vi "FestoCPX.Station.Prod.DropNOK.vi"(7 "prev status":T1=enum."Error", 8 "error in":errorcluster, 10 "Serial":i32, 11 "Slot":T3) -> (0 "error out":errorcluster, 1 "Pause status":T2, 2 "Final status":T1)   [LabVIEW 2016]
uses:
  Station/Station.ProductSlot.ctl
  Sequence/Sequence.Step.Status.ctl
  Sequence/Sequence.Test.BreakReason.ctl
  tools/Translator/Translator.Message.ctl
  tools/EventLog/EventLog.EventSource.ctl
  Station/Station.ValvePosition.ctl
  tools/EventLog/EventLog.CreateError(single).vi
  tools/EventLog/EventLog.New(array).vi
  Sequence/Sequence.SerialsFglb.Action.ctl
  Sequence/Sequence.SerialsFglb.SerialData.ctl
  Global/ApplicationGlobal.vi
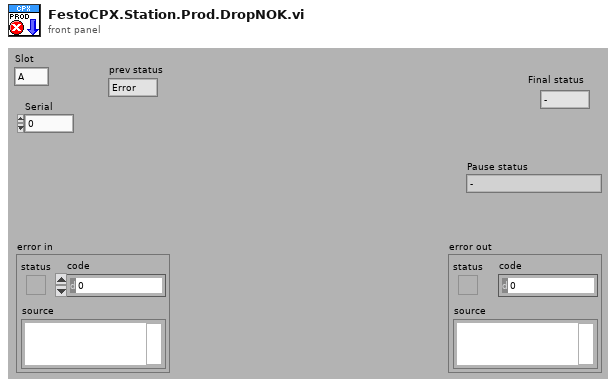
[diagram p1: front panel]
types:
  T1 = typedef "Sequence.Step.Status.ctl" = enum16{"-", "Pending", "Running", "Skipped", "Passed", "Failed", "Done", "Error", "Aborted", "Stopped"}
  T2 = typedef "Sequence.Test.BreakReason.ctl" = enum16{"-", "NOK container", "OK container", "Rev empty", "Rev missing", "Rev wrong", "Fork missing", "Fork wrong", "NOK limit", "Unload failure", "Single slot", "Part done", "Err: Prod move work", "Err: Prod move home", "Err: Prod lift work", "Err: Prod lift home", "Err: Prod Arm Work", "Err: Prod Arm NOK", "Err: Prod Arm OK", "Err: Prod NOK suck", "Err: Prod NOK drop", "Err: Prod OK missing", "Err: Prod OK suck", "Err: Prod OK drop"}
  T3 = typedef "Station.ProductSlot.ctl" = enum8{"A", "B"}
  T4 = typedef "Translator.Message.ctl" = enum16{"-", "Event confirmed", "Log out", "Log in", "Shutdown", "Cancel", "Start", "Begin time", "End time", "Duration", "Service Mode", "Ignore Results", "Serial Format", "On", "Off", "OK", "NOK", "NOK %s", "Home", "Work", "Close", "Open", "In progress...", "Missing", "Empty", "Hardware failure", "Initial", "Default", "Total", "Out of range", "Free disk space is below 1GB - contact technician", "Error %d >> %s", "Error %d >> %s >> %s", "Msg %d >> %s", "Laser msg %d %s", "Laser cmd error %s %d", "Laser cmd failed %s", "Laser cmd warning %s", "Laser disconnected", "Laser status %s", "Laser already started", "Laser job unkonwn %s", "Laser job missing %s", "Laser job select failure %s", "Unable to start laser printing (%s)", "Unable to stop laser printing (%s)", "Laser marking aborted", "Laser marking timeout", "Unable to reset Laser Interlock (%s)", "Unable to trigger Laser. Laser not ready (%s)", "Laser job '%s' coordinates not configured", "Starting %s", "Quitting %s", "Configured", "Initializing", "Quitting", "Loading", "Loaded %d results", "Loaded %d events", "Running", "Stopped", "Summary", "Laser", "Do you want to continue?", "Do you want to delete the configuration?", "The configuration is being used by an order. Unable to delete!", "Press confirm button", "Station is not based. Do you want to exit?", "Station requires changeover. Do you want to run the test?", "Test options are not set as default. Do you want to continue?", "Formatting of WabcoNo is disabled. Do you want to continue?", "Product not detected. Do you want to continue?", "Product scan failed. Do you want to continue?", "Calibration", "Log out?", "System", "All", "IDLE", "Translating...%s", "Not found", "Alarm %s", "Run", "Skip", "Abort", "Repeat", "Please wait...", "Database disconnected", "Database disconnected - changeover disabled!", "Login to database successful", "Login to database failed: %d; %s", "Unable to check the product status of reference %d - database disconnected", "Unable to set the product status of reference %d - database disconnected", "Variant file backup %s", "Read variant (%s)", "Result", "Station armed!", "Station requires changeover!", "Select reference number...", "EMERGENCY BUTTON - press Control button", "EMERGENCY DOOR - press Control button", "Resetting Emergency...", "Unable to reset safety circuit - Emergency Button pressed", "Unable to reset safety circuit - Emergency Side Door open", "Station not based", "Station based", "Station not empty", "Station basing...", "No order", "Press Start to begin new order", "Scanning new order", "Order NOK. Correct or scan again", "Order OK. Press Accept", "Order ready", "Revolver incorrect", "Fork incorrect", "Revolver missing", "Revolver empty", "Container missing", "Offline results", "Offline statistics", "Updating statistics %.1f %%", "DMC Configurator", "Door open", "Close the front door", "Press start button", "Done. Open the front door", "Running...", "Running...%.1f %%", "Pause %s", "Pause %s. NOK container missing", "Pause %s. OK container missing", "Pause %s. Revolver empty", "Pause %s. Revolver missing", "Pause %s. Revolver incorrect", "Pause %s. Fork missing", "Pause %s. Fork incorrect", "Pause %s. Too many failures", "Pause %s. Unloading failure", "Pause %s. One slot is not working", "Pause %s. Part order is done. Empty OK container", "Pause %s. Unable to move product to slot", "Pause %s. Unable to move back product pusher", "Pause %s. Unable to lift product", "Pause %s. Unable to move back product lifter", "Pause %s. Unable to move product arm to Work", "Pause %s. Unable to move product arm to NOK", "Pause %s. Unable to move product arm to OK", "Pause %s. Unable to unsuck the NOK product", "Pause %s. Unable to drop the NOK product", "Pause %s. Product OK missing", "Pause %s. Unable to unsuck the OK product", "Pause %s. Unable to drop the OK product", "Stopping...", "File '%s' is missing", "File '%s' is broken", "File '%s' is running", "Log file started (%s)", "Log file ended (%s)", "Log file stopped (%s)", "Log file ignored (%s)", "Log file exported (%s)", "Log file export failed (%s)", "Wrong serial number in log file", "Wrong reference number in log file", "Test steps are missing", "%s = %.3f", "Process param '%s' not found in DB", "Process param '%s' wrong order", "Process param '%s' value %.3f out of limits (%.3f; %.3f)", "Step%d param '%s' not found in DB", "Step%d param '%s' wrong order", "Step%d param '%s' value %.3f out of limits (%.3f; %.3f)", "Step%d EV '%s' not found in DB", "Step%d EV '%s' wrong order", "\"%s\" not found in DB", "\"%s\" wrong order", "\"%s\" value %.3f out of limits (%.3f; %.3f)", "\"%s\" not found in software", "Process init (%s)", "Process started", "Process restarted", "Process run", "Process done", "Process done - remove OK container", "Process aborted", "Process aborted at work", "Process aborted at home", "Process error", "Process error at home", "Process error at work", "Process close", "Process pause", "Process continue", "Process door open", "Process door close", "Process pause at slot %s due to %s", "Select plate from the order to process", "Do you want to start the process?", "Do you want to continue the process?", "There is unfinished order. Do you want to put the new order?", "Product %s %d OK", "Product %s %d NOK", "Unable to unload the slot %s. Product missing in the slot", "Unable to unload the slot %s. Product already in the arm", "Unable to accept the product as OK. Product missing in slot %s", "Unable to accept the product as OK. Product could not drop into the container at slot %s", "Unable to accept the product as NOK. Product could not drop into the container at slot %s", "Scan failed. Error %s", "Scan failed. Scanner disconnected", "Scan failed. Wrong Wabco number %d, limit (%d,%d)", "Scan failed. Wrong serial number %d, limit (%d,%d)", "Scan failed. Wrong date %d, limit (%d,%d)", "Scan failed. Wrong product wabco number %d (expected %d)", "Scan failed. Wrong product serial number %d (expected > 0)", "Scan OK %s", "Scan failed. Unable to determine table position (%s)", "Scan failed. Timeout", "Tune failed. Scanner disconnected", "Tune failed. Timeout", "%s = %d", "%s = %d->%d", "Unable to set %s = %.2f - Air Pressure Inside off", "Unable to set digital output '%s' = %d", "Unable to activate air pressure inside - timeout", "Unable to activate air pressure inside - aborted", "Unable to switch on Air Main Valve - Air Pressure Inlet off", "Unable to switch on Air Main Valve - Door open", "Unable to switch off Air Main Valve - timeout", "Unable to switch off Air Main Valve - aborted", "Unable to rotate Table - timeout", "Unable to rotate Table - aborted", "Unable to rotate Table - Product Move not in Home position", "Unable to rotate Table - Air Pressure Inside off", "Unable to rotate Table - Product Lift A not in Home position", "Unable to rotate Table - Product Lift B not in Home position", "Unable to rotate Table - unlock before movement timeout", "Unable to rotate Table - lock after movement timeout", "Unable to move Table Lock to %s position - timeout", "Unable to move Table Lock to %s position - aborted", "Unable to move Table Lock to %s position - Air Pressure Inside off", "Unable to move Table Lock to %s position - Table not in position", "Unable to move Product Lift A to %s position - timeout", "Unable to move Product Lift B to %s position - timeout", "Unable to move Product Lift A to %s position - aborted", "Unable to move Product Lift B to %s position - aborted", "Unable to move Product Lift A to %s position - Air Pressure Inside off", "Unable to move Product Lift B to %s position - Air Pressure Inside off", "Unable to move Product Lift A to %s position - Table not locked", "Unable to move Product Lift B to %s position - Table not locked", "Unable to move Product Lift A to %s position - Product Arm not in Work position", "Unable to move Product Lift B to %s position - Product Arm not in Work position", "Unable to set Product Suction Gripper %s to %s - timeout", "Unable to set Product Suction Gripper %s to %s - aborted", "Unable to set Product Suction Gripper %s to %s - Air Pressure Inside off", "Unable to set Product Suction Gripper %s to %s - Table slot unkown", "Unable to move Product Arm to %s position - timeout", "Unable to move Product Arm to %s position - aborted", "Unable to move Product Arm to %s position - Air Pressure Inside off", "Unable to move Product Arm to %s position - Product Lift A not in Home position", "Unable to move Product Arm to %s position - Product Lift B not in Home position", "Unable to move Product to %s position - timeout", "Unable to move Product to %s position - aborted", "Unable to move Product to %s position - Air Pressure Inside off", "Unable to move Product to %s position - Table not in position"}
  T5 = typedef "EventLog.EventSource.ctl" = enum16{"All", "Gui", "Ref", "File", "Arch", "Seq", "CPX", "DB", "Laser", "Scan.P", "Scan.O"}
  T6 = typedef "Station.ValvePosition.ctl" = enum16{"Home", "Work"}
  T7 = typedef "FestoCPX.Station.ProdPresent.ctl" = cluster{"Slot1":cluster{"A":bool, "B":bool}, "Slot2":cluster{"A":bool, "B":bool}, "Slot3":cluster{"A":bool, "B":bool}, "Slot4":cluster{"A":bool, "B":bool}, "Final":cluster{"A":bool, "B":bool}, "OK":cluster{"A":bool, "B":bool}, "Container":cluster{"OK":bool, "NOK":bool}}
  T8 = typedef "Sequence.SerialsFglb.SerialData.ctl" = cluster{"TS":timestamp, "Slot":T3, "Serial":i32, "Global":bool}
  T9 = typedef "Sequence.SerialsFglb.Action.ctl" = enum16{"init", "get", "get next", "pass", "fail", "confirm", "clean"}
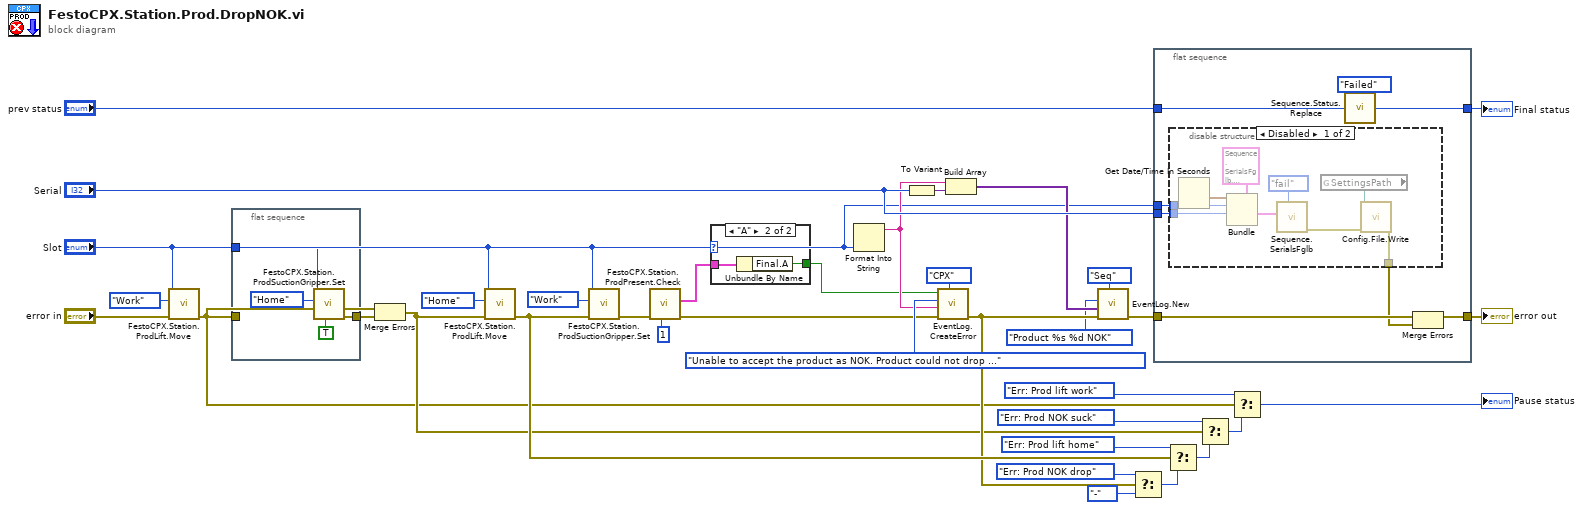
[diagram p0: block diagram]
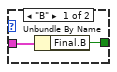
[diagram p3: hidden frame]
diagram:
  n1 = call "FestoCPX.Station.ProdLift.Move.vi"("error in"="error in", "Position"=Station.ValvePosition."Work", "Slot"="Slot") -> ("error out"=w3:errorcluster)  [unwired: 8 in]
  n2 = flat-sequence {
    tunnel: w3 -> [_]
    tunnel: [w38] -> w14
    tunnel: "Slot" -> [w37]
    frame #0 {
      n3 = call "FestoCPX.Station.ProdSuctionGripper.Set.vi"("wait for product (F)"=TRUE, "Position"=Station.ValvePosition."Home", "Slot"=w37) -> ("error out"=w38:errorcluster)  [unwired: 7 in, 1 out]
    }
  }
  n4 = Merge Errors(w3, w14) -> (w4:errorcluster)
  n5 = call "FestoCPX.Station.ProdLift.Move.vi"("error in"=w4, "Position"=Station.ValvePosition."Home", "Slot"="Slot") -> ("error out"=w13:errorcluster)  [unwired: 8 in]
  n6 = call "FestoCPX.Station.ProdSuctionGripper.Set.vi"("error in"=w13, "Position"=Station.ValvePosition."Work", "Slot"="Slot") -> ("error out"=w22:errorcluster)  [unwired: 7 in, 1 out]
  n7 = call "FestoCPX.Station.ProdPresent.Check.vi"("Stab Counter (0)"=1 ("Max Stab time [ms] (0)"), "error in"=w22) -> ("error out"=w26:errorcluster, "Prod Present"=w32:T7)  [unwired: 4 in, 4 out]
  n8 = case shown="\"A\"" "Slot" {
    tunnel: w32 -> [w42 w44]
    tunnel: [w41 w43] -> w9
    frame "B" {
      n9 = Unbundle By Name(w42) -> ("Final.B"=w41:bool)
    }
    frame "A" {
      n10 = Unbundle By Name(w44) -> ("Final.A"=w43:bool)
    }
  }
  n11 = Format Into String("Slot") -> (resulting string=w28:string)  [unwired: 3 in, 1 out]
  n12 = To Variant(anything="Serial") -> (Variant=w30:variant)
  n13 = call-poly "EventLog.CreateError.vi"("Source (All)"=EventLog.EventSource."CPX", "error in"=w26, "arg"=w28, "msg"=Translator.Message."Unable to accept the product as NOK. Product could not drop into the container at slot %s", "create (T)"=w9) -> ("error out"=w12:errorcluster)  [unwired: 6 in]
  n14 = Build Array(w28, w30) -> (w29:variant[])
  n15 = call-poly "EventLog.New.vi"("Source (All)"=EventLog.EventSource."Seq", "error in (no error)"=w12, "Arguments"=w29, "Message (-)"=Translator.Message."Product %s %d NOK" ("msg")) -> ("error out"=w6:errorcluster)  [unwired: 6 in, 1 out]
  n16 = Select(t=Sequence.Test.BreakReason."Err: Prod NOK drop" ("A.pause"), s=w12, f=Sequence.Test.BreakReason."-") -> (s? t:f=w16:T2)
  n17 = flat-sequence {
    tunnel: "Serial" -> [w52]
    tunnel: [w45] -> w8
    tunnel: "Slot" -> [w51]
    tunnel: w6 -> [w50]
    tunnel: [w49] -> w5
    tunnel: "prev status" -> [w46]
    frame #0 {
      n18 = disable-structure shown="Disabled" {
        disable-tunnel: w52 -> [w61 _]
        disable-tunnel: w51 -> [w60 _]
        disable-tunnel: [w53 _] -> w48
        frame Disabled {
          n19 = Get Date/Time In Seconds() -> (seconds since 1Jan1904=w58:timestamp)
          n20 = Bundle(cluster=T8 {"TS"=timestamp(0 s since 1904-01-01), "Slot"=enum."A", "Serial"=0, "Global"=FALSE} ("SerialData"), "TS"=w58, "Slot"=w60, "Serial"=w61) -> (w56:T8)  [unwired: 1 in]
          n21 = call "Sequence.SerialsFglb.vi"("Action (get)"=Sequence.SerialsFglb.Action."fail" ("Action"), "Serial data in"=w56) -> ("error out"=w54:errorcluster)  [unwired: 5 in, 4 out]
          n22 = global read "ApplicationGlobal.vi" "SettingsPath"() -> (w55:path)
          n23 = call "Config.File.Write.vi"("error in"=w54, "path"=w55) -> ("error out"=w53:errorcluster)  [unwired: 9 in]
        }
        frame Enabled {
        }
      }
      n24 = call "Sequence.Status.Replace.vi"("old status"=w46, "new status (Done)"=Sequence.Step.Status."Failed" ("t")) -> ("status out"=w45:T1)
      n25 = Merge Errors(w50, w48) -> (w49:errorcluster)
    }
  }
  n26 = Select(t=Sequence.Test.BreakReason."Err: Prod lift home" ("A.pause"), s=w13, f=w16) -> (s? t:f=w18:T2)
  n27 = Select(t=Sequence.Test.BreakReason."Err: Prod NOK suck" ("A.pause"), s=w4, f=w18) -> (s? t:f=w24:T2)
  n28 = Select(t=Sequence.Test.BreakReason."Err: Prod lift work" ("A.pause"), s=w3, f=w24) -> (s? t:f=→"Pause status":T2)
  "error out" <- w5
  "Final status" <- w8
